vi "WFS_Thorlabs_testPanel.vi"() -> ()   [LabVIEW 2016]
uses:
  Type definitions/WFS cam and pupil config.ctl
  Type definitions/WFS wavefront and Zernike fit.ctl
  Type definitions/WFS wavefront data.ctl
  Type definitions/States enum in WFS_Thorlabs_testPanel.ctl
  <vilib>/Analysis/5stat.llb/RMS (DBL).vi
  <vilib>/Analysis/baseanly.llb/Mean (DBL).vi
  <vilib>/Platform/NI_3dgraph.lvlib
  <vilib>/Analysis/NI_AALBase.lvlib
  <vilib>/Analysis/NI_AALPro.lvlib
panel:
  in  "Rolling average, frames":i32=10 caption="Average Count" min=1 max=255 step=1
  in  "Output":enum32{"Graphical output", "Numerical"}(tab)
  in  "Measured WF":refnum<k7>(container)
  out "Zernike coeffs":dbl[](graph)
  in  "Fitting errors":refnum<k7>(container)
  out "WF data":T1
  out "Rad. of curvature (mm)":dbl
  out "error out":errorcluster
  out "spots_y":i32
  out "spots_x":i32
  out "Exp Time Incr":dbl=0.0554 caption="Exposure Time Incr"
  out "Exp time Max, ms":dbl=66.6147666666 caption="Exposure Time Max"
  out "Exp time Min, ms":dbl=0.07936666666666665 caption="Exposure Time Min"
  in  "stop":bool
  out "Ambient light":string
  out "Light power":string
  in  "WF and Zernike fit config":T2={"Limit meas. to pupil"=1, "Cancel WF tilt"=enum."Yes", "Zern. order max."=5, "wavelength, um"=0.633} {"wavelength, um" format="%.3f"; "Limit meas. to pupil" items=["Yes"=1, "No"=0]}
  in  "WFS cam & pupil config":T3={"Trigger Mode"=enum."Continuous", "Auto exposure"=TRUE, "Exposure time (ms)"=0.07936666666666667, "Master gain"=1.0, "Cam img size"=1, "Pupil diam X (mm)"=4.5, "Pupil diam Y (mm)"=4.5} {"Cam img size" items=["1280x1024 = 5.95x4.76mm", "1024x1024 = 4.76x4.76mm", "768x768 = 3.57x3.57mm", "512x512 = 2.38x2.38mm", "320x320 = 1.49x1.49mm"]; "Exposure time (ms)" min=0.0793667 max=66.6148 step=0.0554 format="%#.6f"}
  in  "error in":errorcluster
  out "InstName":string caption="Instrument Name"
  # "Shack-Hartmann wavefront sensor config"
  # "All units are lambda (wavelength)"
  # "For Shack-Hartmann sensor models:\nThorlabs WFS-150, WFS-300, WFS-20"
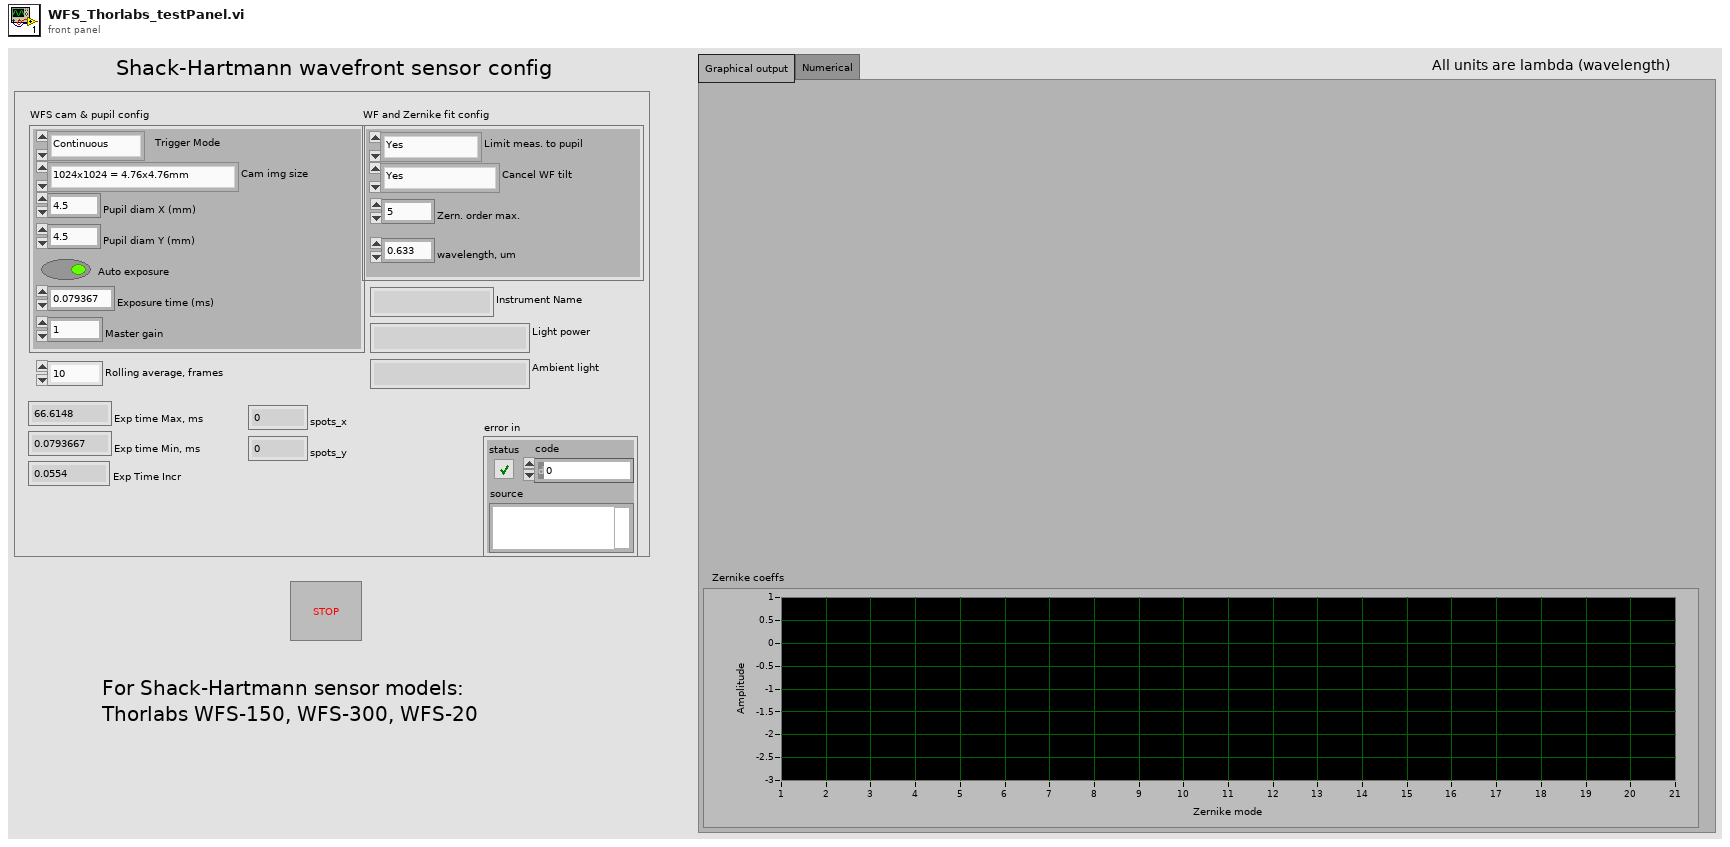
[diagram p1: front panel]
types:
  T1 = typedef "WFS wavefront data.ctl" = cluster{"ArrayWF":sgl[][], "ArrayZernike":sgl[], "WF_PV":dbl, "WF_RMS":dbl, "FittingErrors":dbl[][], "Error_mean":dbl, "Error_RMS":dbl}
  T2 = typedef "WFS wavefront and Zernike fit.ctl" = cluster{"Limit meas. to pupil":i32, "Cancel WF tilt":enum16{"No", "Yes"}, "Zern. order max.":i32, "wavelength, um":dbl}
  T3 = typedef "WFS cam and pupil config.ctl" = cluster{"Trigger Mode":enum16{"Continuous", "Slope H->L", "Slope L->H", "Software"}, "Auto exposure":bool, "Exposure time (ms)":dbl, "Master gain":dbl, "Cam img size":i32, "Pupil diam X (mm)":dbl, "Pupil diam Y (mm)":dbl}
  T4 = typedef "States enum in WFS_Thorlabs_testPanel.ctl" = enum16{"Initialize", "Configure", "Measure", "Stop", "Exit", "Health check"}
  T5 = enum16{"Initialize", "Configure", "Measure", "Stop", "Exit"}
  T6 = enum16{"Initialize", "Configure", "Measure", "Stop", "Exit", "Health check"}
  T7 = enum16{"Continuous", "Slope H->L", "Slope L->H", "Software"}
  T8 = cluster{"ArrayWF":dbl[][], "ArrayZernike":dbl[], "WF_PV":dbl, "WF_RMS":dbl, "FittingErrors":dbl[][], "Error_mean":dbl, "Error_RMS":dbl}
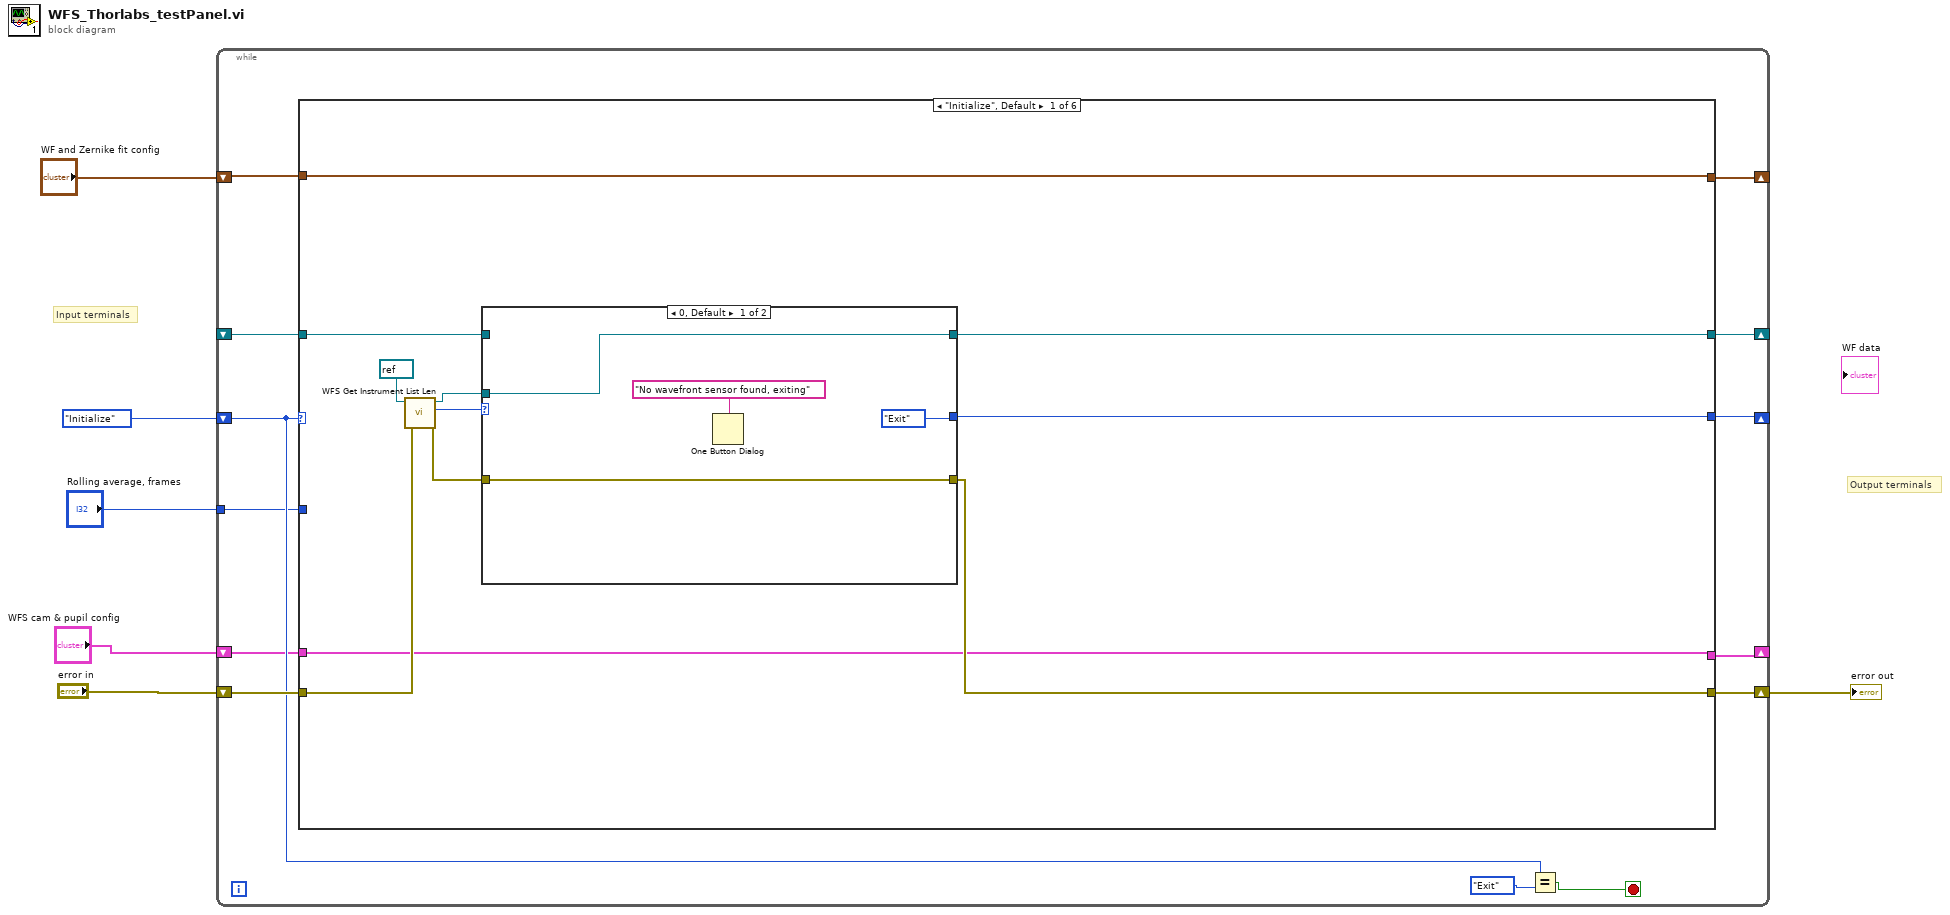
[diagram p0: block diagram]
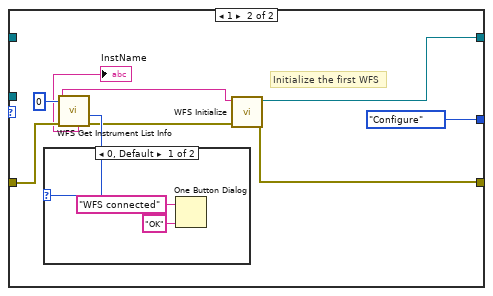
[diagram p2: hidden frame]
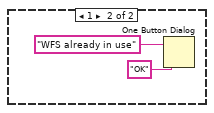
[diagram p3: hidden frame]
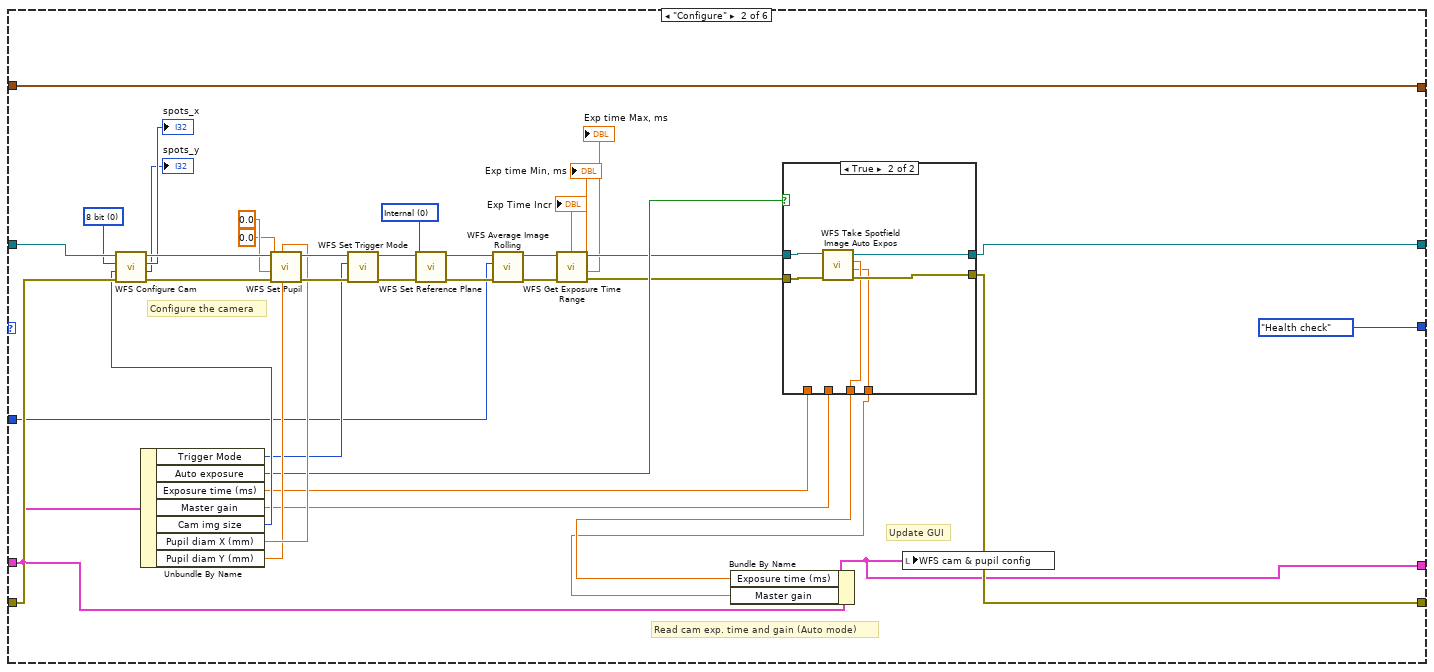
[diagram p4: hidden frame]
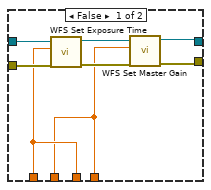
[diagram p5: hidden frame]
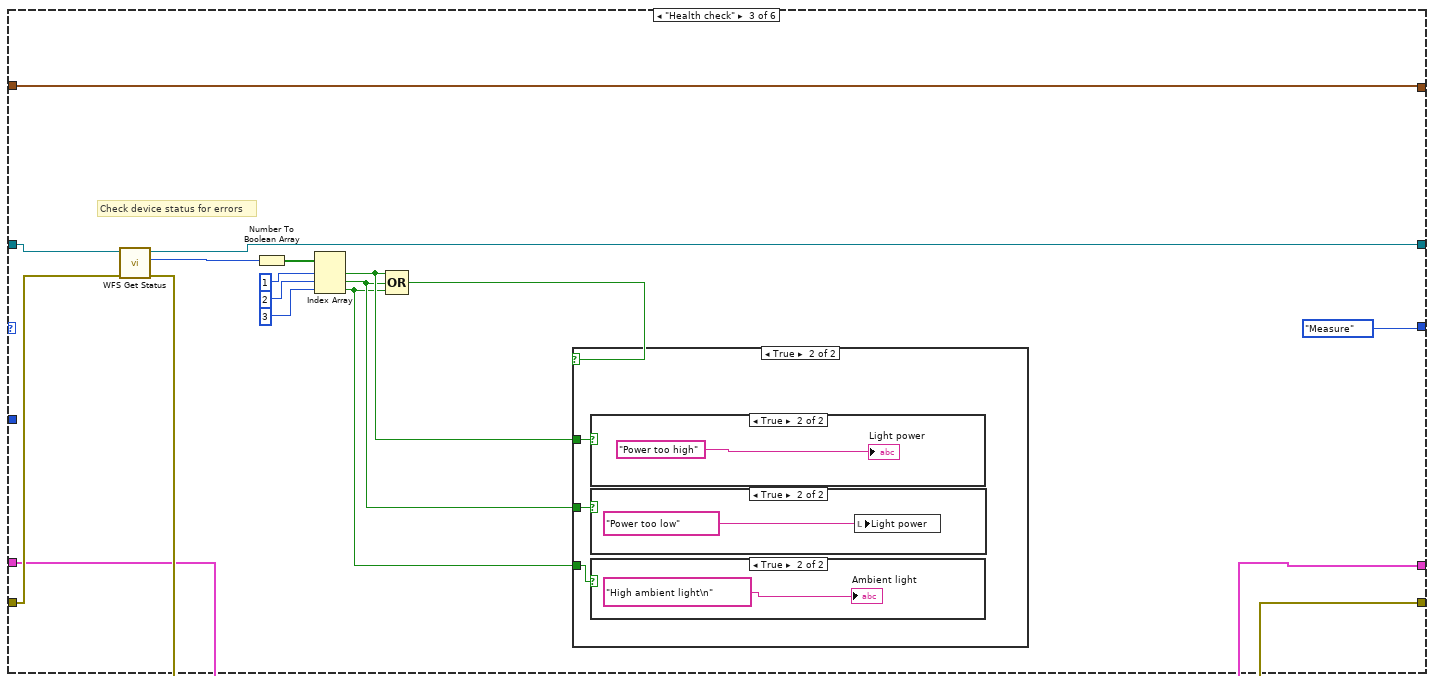
[diagram p6: hidden frame]
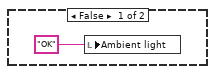
[diagram p8: hidden frame]
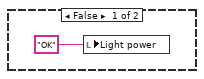
[diagram p9: hidden frame]
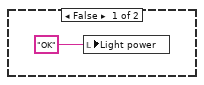
[diagram p10: hidden frame]
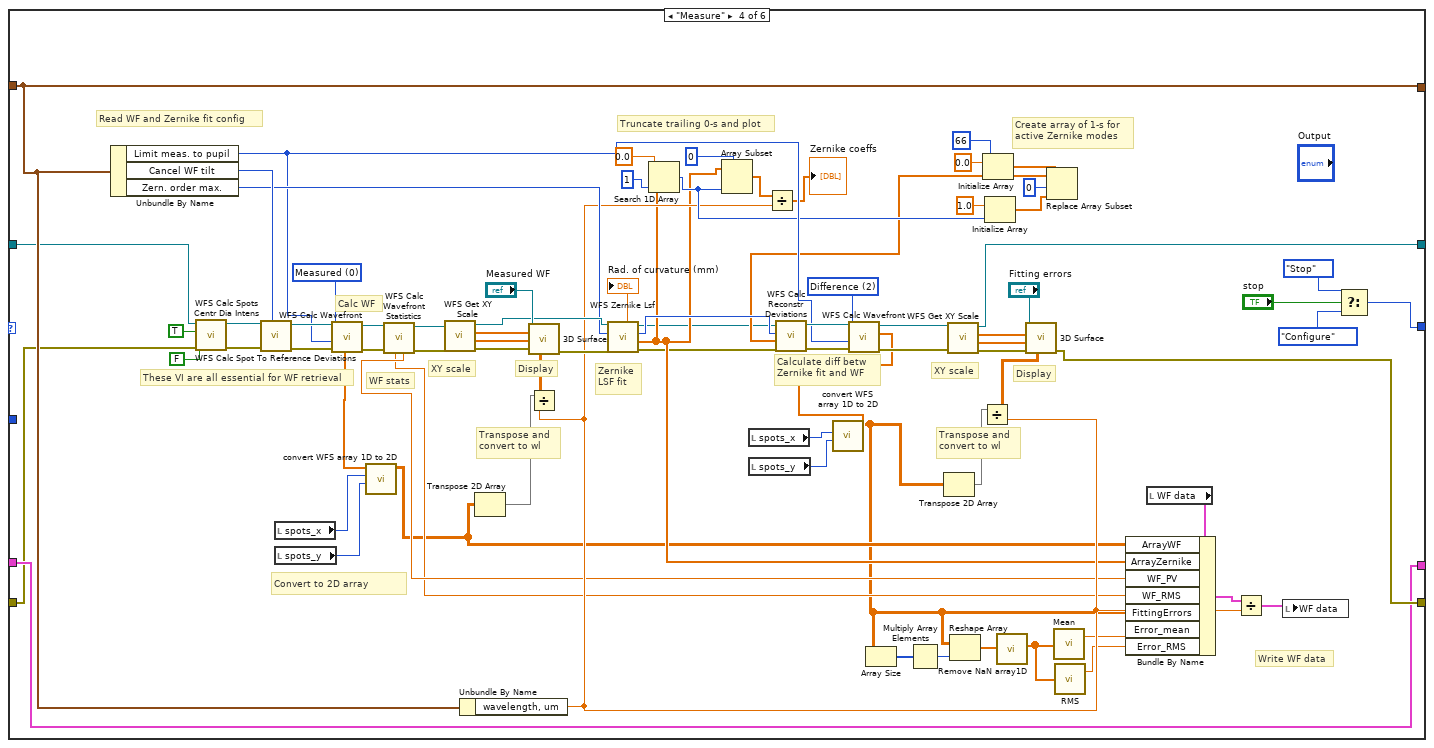
[diagram p11: hidden frame]
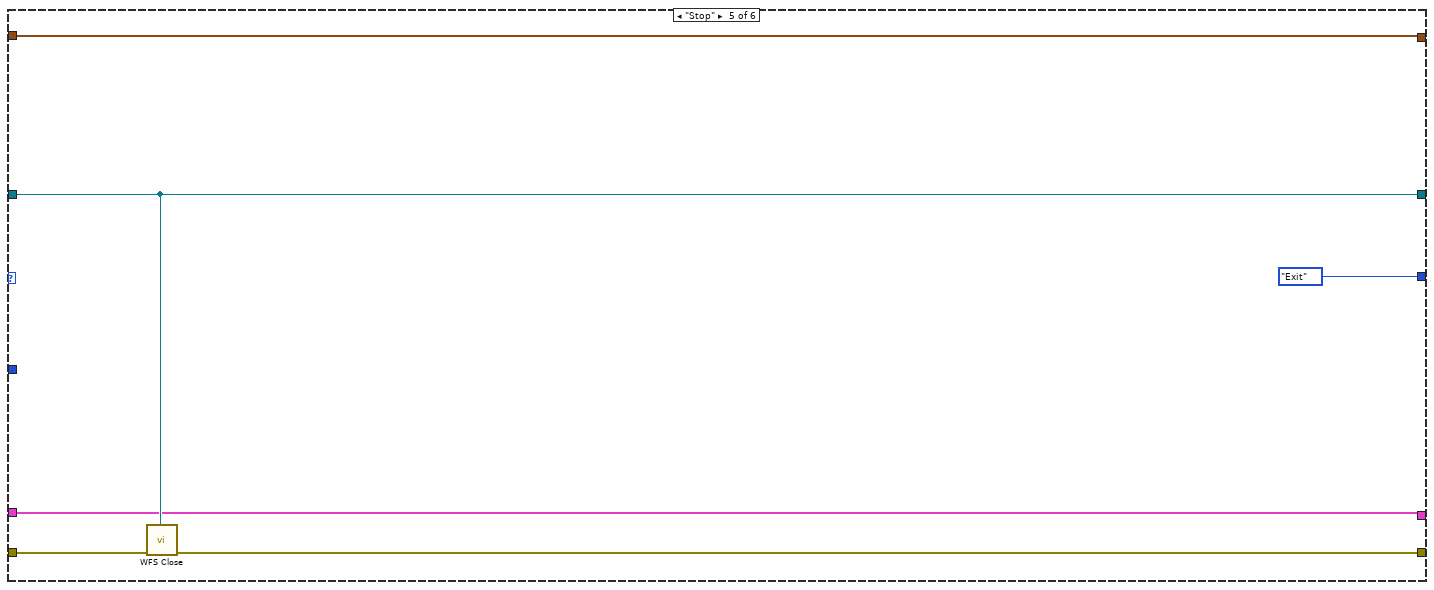
[diagram p12: hidden frame]
diagram:
  # "Input terminals"
  # "Output terminals"
  n1 = while {
    shift-right: [w18] -> w2
    shift-left: "error in" -> [w19]
    shift-right: [w17] -> _
    shift-left: _ -> [w16]
    shift-right: [w15] -> _
    shift-left: States_enum_in_WFS_Thorlabs_testPanel."Initialize" -> [w14]
    shift-right: [w10] -> _
    shift-left: "WFS cam & pupil config" -> [w11]
    shift-right: [w8] -> _
    shift-left: "WF and Zernike fit config" -> [w9]
    tunnel: "Rolling average, frames" -> [w7]
    stop <- w13 stop-if-true
    n2 = case shown="\"Initialize\", Default" w14 {
      selector: w14 -> [_ _ _ _ _ w213]
      tunnel: w19 -> [w30 w85 w111 w127 w211 w215]
      tunnel: [w26 w79 w104 w171 w210 w215] -> w18
      tunnel: [w25 w80 w109 w174 w212 w216] -> w17
      tunnel: w16 -> [w24 w86 w112 w126 w212 w216]
      tunnel: [w21 T6."Health check" T5."Measure" w189 T6."Exit" w213] -> w15
      tunnel: w11 -> [w23 w65 w103 w128 w209 w214]
      tunnel: [w23 w64 w103 w128 w209 w214] -> w10
      tunnel: w9 -> [w22 w56 w102 w157 w208 w217]
      tunnel: [w22 w56 w102 w157 w208 w217] -> w8
      tunnel: w7 -> [_ w48 _ _ _ _]
      frame "Initialize", Default {
        n3 = call "WFS Get Instrument List Len.vi"("error in (no error)"=w30, "instrument handle"=refnum<visa-resource-name> refnum) -> ("error out"=w27:errorcluster, "Instrument Count"=w28:i32, "instrument handle out"=w20:refnum<visa-resource-name>)  [unwired: 7 in]
        n4 = case shown="0, Default" w28 {
          tunnel: [w33 w38] -> w26
          tunnel: w27 -> [w33 w42]
          tunnel: [w31 w39] -> w25
          tunnel: w24 -> [_ _]
          tunnel: [T5."Exit" T5."Configure"] -> w21
          tunnel: w20 -> [w31 _]
          frame 0, Default {
            n5 = One Button Dialog(message="No wavefront sensor found, exiting") -> ()  [unwired: 1 in, 1 out]
          }
          frame 1 {
            # "Initialize the first WFS"
            n6 = call "WFS Get Instrument List Info.vi"("error in (no error)"=w42, "Instrument List Index"=0) -> ("error out"=w40:errorcluster, "In Use"=w41:i32, "Instrument Name"=→"InstName":string, "Resource Name"=w37:string)  [unwired: 3 in, 3 out]
            n7 = case shown="0, Default" w41 {
              frame 0, Default {
                n8 = One Button Dialog(message="WFS connected", button name ("OK")="OK") -> ()  [unwired: 1 out]
              }
              frame 1 {
                n9 = One Button Dialog(message="WFS already in use", button name ("OK")="OK") -> ()  [unwired: 1 out]
              }
            }
            n10 = call "WFS Initialize.vi"("error in (no error)"=w40, "resource name"=w37) -> ("error out"=w38:errorcluster, "instrument handle out"=w39:refnum<visa-resource-name>)  [unwired: 8 in]
          }
        }
      }
      frame "Configure" {
        w73 = 0 items=["Internal", "User"] ("Reference Index (Internal)")
        w76 = 0 items=["16 bit"=1, "8 bit"=0] ("Pixel Format (8 bit)")
        # "Update GUI"
        # "Read cam exp. time and gain (Auto mode)"
        # "Configure the camera"
        n11 = Unbundle By Name(w65) -> ("Trigger Mode"=w69:T7, "Auto exposure"=w68:bool, "Exposure time (ms)"=w67:dbl, "Master gain"=w66:dbl, "Cam img size"=w72:i32, "Pupil diam X (mm)"=w71:dbl, "Pupil diam Y (mm)"=w70:dbl)
        n12 = call "WFS Configure Cam.vi"("error in (no error)"=w85, "Cam Resol. Index (1280x1024      640x480      1440x1080)"=w72, "Pixel Format (8 bit)"=w76, "instrument handle"=w86) -> ("error out"=w84:errorcluster, "Spots Y"=→"spots_y":i32, "Spots X"=→"spots_x":i32, "instrument handle out"=w83:refnum<visa-resource-name>)  [unwired: 4 in]
        n13 = call "WFS Set Pupil.vi"("Pupil Diameter Y mm"=w70, "Pupil Diameter X mm"=w71, "error in (no error)"=w84, "Pupil Center Y mm"=0.0, "Pupil Center X mm"=0.0, "instrument handle"=w83) -> ("error out"=w81:errorcluster, "instrument handle out"=w82:refnum<visa-resource-name>)  [unwired: 4 in]
        n14 = call "WFS Set Trigger Mode.vi"("error in (no error)"=w81, "Trigger Mode"=w69, "instrument handle"=w82) -> ("error out"=w74:errorcluster, "instrument handle out"=w75:refnum<visa-resource-name>)  [unwired: 7 in]
        n15 = call "WFS Set Reference Plane.vi"("error in (no error)"=w74, "Reference Index (Internal)"=w73, "instrument handle"=w75) -> ("error out"=w49:errorcluster, "instrument handle out"=w50:refnum<visa-resource-name>)  [unwired: 7 in]
        n16 = call "WFS Average Image Rolling.vi"("error in (no error)"=w49, "Average Count"=w48, "instrument handle"=w50) -> ("error out"=w51:errorcluster, "instrument handle out"=w52:refnum<visa-resource-name>)  [unwired: 7 in]
        n17 = call "WFS Get Exposure Time Range.vi"("error in (no error)"=w51, "instrument handle"=w52) -> ("error out"=w60:errorcluster, "Exposure Time Max"=→"Exp time Max, ms":dbl, "Exposure Time Min"=→"Exp time Min, ms":dbl, "instrument handle out"=w61:refnum<visa-resource-name>, "Exposure Time Incr"=→"Exp Time Incr":dbl)  [unwired: 5 in]
        n18 = case shown="True" w68 {
          tunnel: [w92 w100] -> w80
          tunnel: [w91 w99] -> w79
          tunnel: w60 -> [w90 w97]
          tunnel: w61 -> [w89 w98]
          tunnel: w67 -> [w88 _]
          tunnel: w66 -> [w87 _]
          tunnel: [w88 w96] -> w63
          tunnel: [w87 w95] -> w62
          frame False {
            n19 = call "WFS Set Exposure Time.vi"("error in (no error)"=w90, "Exposure Time Set"=w88, "instrument handle"=w89) -> ("error out"=w94:errorcluster, "instrument handle out"=w93:refnum<visa-resource-name>)  [unwired: 6 in, 1 out]
            n20 = call "WFS Set Master Gain.vi"("error in (no error)"=w94, "Master Gain Set"=w87, "instrument handle"=w93) -> ("error out"=w91:errorcluster, "instrument handle out"=w92:refnum<visa-resource-name>)  [unwired: 6 in, 1 out]
          }
          frame True {
            n21 = call "WFS Take Spotfield Image Auto Expos.vi"("error in (no error)"=w97, "instrument handle"=w98) -> ("error out"=w99:errorcluster, "Master Gain Act"=w95:dbl, "Exposure Time Act"=w96:dbl, "instrument handle out"=w100:refnum<visa-resource-name>)  [unwired: 6 in]
          }
        }
        n22 = Bundle By Name(cluster=w65, "Exposure time (ms)"=w63, "Master gain"=w62) -> (w64:T3)
        n23 = local write "WFS cam & pupil config"(w64) -> ()
      }
      frame "Health check" {
        # "Check device status for errors"
        n24 = call "WFS Get Status.vi"("error in (no error)"=w111, "instrument handle"=w112) -> ("error out"=w104:errorcluster, "Device Status"=w110:i32, "instrument handle out"=w109:refnum<visa-resource-name>)  [unwired: 7 in]
        n25 = Number To Boolean Array(number=w110) -> (Boolean array=w113:bool[])
        n26 = Index Array(array=w113, index #1=1 ("index"), index #2=2 ("index"), index #3=3 ("index")) -> (element #1=w107:bool, element #2=w106:bool, element #3=w105:bool)
        n27 = Compound Arithmetic op=OR(w107, w106, w105) -> (w108:bool)
        n28 = case shown="True" w108 {
          tunnel: w107 -> [_ w119]
          tunnel: w106 -> [_ w118]
          tunnel: w105 -> [_ w117]
          frame False {
          }
          frame True {
            n29 = case shown="True" w119 {
              frame False {
                n30 = local write "Light power"("OK" ("Device Status")) -> ()
              }
              frame True {
                "Light power" <- "Power too high"
              }
            }
            n31 = case shown="True" w118 {
              frame False {
                n32 = local write "Light power"("OK" ("Device Status")) -> ()
              }
              frame True {
                n33 = local write "Light power"("Power too low") -> ()
              }
            }
            n34 = case shown="True" w117 {
              frame False {
                n35 = local write "Ambient light"("OK" ("Device Status 2")) -> ()
              }
              frame True {
                "Ambient light" <- "High ambient light\n"
              }
            }
          }
        }
      }
      frame "Measure" {
        w180 = 2 items=["Measured", "Reconstructed", "Difference"] ("Wavefront Type (Measured)")
        w185 = 0 items=["Measured", "Reconstructed", "Difference"] ("Wavefront Type (Measured)")
        # "Create array of 1-s for \nactive Zernike modes"
        # "Truncate trailing 0-s and plot"
        # "Transpose and \nconvert to wl"
        # "Transpose and \nconvert to wl"
        # "Convert to 2D array"
        # "Display"
        # "XY scale"
        # "Calculate diff betw \nZernike fit and WF"
        # "Write WF data"
        # "Calc WF"
        # "XY scale"
        # "WF stats"
        # "Display"
        # "Read WF and Zernike fit config"
        # "These VI are all essential for WF retrieval"
        # "Zernike \nLSF fit"
        n36 = Unbundle By Name(w157) -> ("Limit meas. to pupil"=w179:i32, "Cancel WF tilt"=w194:enum16{"No", "Yes"}, "Zern. order max."=w184:i32)
        n37 = call "WFS Calc Spots Centr Dia Intens.vi"("error in (no error)"=w127, "Calculate Diameters (Off)"=FALSE, "Dynamic Noise Cut (On)"=TRUE, "instrument handle"=w126) -> ("error out"=w199:errorcluster, "instrument handle out"=w200:refnum<visa-resource-name>)  [unwired: 6 in]
        n38 = call "WFS Calc Spot To Reference Deviations.vi"("error in (no error)"=w199, "Cancel Wavefront Tilt (No)"=w194, "instrument handle"=w200) -> ("error out"=w198:errorcluster, "instrument handle out"=w197:refnum<visa-resource-name>)  [unwired: 7 in]
        n39 = local read "spots_x"() -> (w141:i32)
        n40 = local read "spots_y"() -> (w140:i32)
        n41 = call "WFS Calc Wavefront.vi"("error in (no error)"=w198, "Limit to Pupil (No)"=w179, "Wavefront Type (Measured)"=w185, "instrument handle"=w197) -> ("error out"=w133:errorcluster, "Array Wavefront"=w142:sgl[], "instrument handle out"=w134:refnum<visa-resource-name>)  [unwired: 5 in]
        n42 = call "convert WFS array 1D to 2D.vi"("spots_y"=w140, "spots_x"=w141, "WF 1D input"=w142) -> ("FW 2D output"=w139:sgl[][])  [unwired: 8 in]
        n43 = call "WFS Calc Wavefront Statistics.vi"("error in (no error)"=w133, "instrument handle"=w134) -> ("error out"=w131:errorcluster, "instrument handle out"=w132:refnum<visa-resource-name>, "Diff"=w150:dbl, "RMS"=w149:dbl)  [unwired: 2 in, 4 out]
        n44 = call "WFS Get XY Scale.vi"("error in (no error)"=w131, "instrument handle"=w132) -> ("error out"=w206:errorcluster, "Array Scale Y"=w204:sgl[], "Array Scale X"=w205:sgl[], "instrument handle out"=w196:refnum<visa-resource-name>)  [unwired: 6 in]
        n45 = Unbundle By Name(w157) -> ("wavelength, um"=w152:dbl)
        n46 = Transpose 2D Array(2D array=w139) -> (transposed array=w187:sgl[][])
        n47 = Divide(x=w187, y=w152) -> (x/y=w186:dbl[][])
        n48 = call <vilib>:"3D Surface.vi"("z matrix"=w186, "error in (no error)"=w206, "y vector"=w204, "x vector"=w205, "3D graph"="Measured WF") -> ("error out"=w195:errorcluster)  [unwired: 5 in, 1 out]
        n49 = call "WFS Zernike Lsf.vi"("error in (no error)"=w195, "Zernike Orders In"=w184, "instrument handle"=w196) -> ("error out"=w129:errorcluster, "Array Zernike um"=w151:sgl[], "Zernike Orders Out"=w183:i32, "instrument handle out"=w130:refnum<visa-resource-name>, "RoC mm"=→"Rad. of curvature (mm)":dbl)  [unwired: 3 in, 1 out]
        n50 = Search 1D Array(1D array=w151, element=sgl 0.0, start index (0)=1) -> (index of element=w161:i32)
        n51 = Array Subset(array=w151, index=0, length=w161) -> (w156:sgl[])
        n52 = local read "spots_x"() -> (w138:i32)
        n53 = local read "spots_y"() -> (w137:i32)
        n54 = Divide(x=w156, y=w152) -> (x/y=→"Zernike coeffs":dbl[])
        n55 = Initialize Array(0.0 ("element"), 66 ("dimension size")) -> (w163:dbl[])
        n56 = Initialize Array(1.0 ("element"), w161) -> (w159:dbl[])
        n57 = Replace Array Subset(array=w163, new element=w159, index=0) -> (w158:dbl[])
        n58 = call "WFS Calc Reconstr Deviations.vi"("error in (no error)"=w129, "Array Zernike Reconstruct"=w158, "Zernike Orders"=w183, "instrument handle"=w130) -> ("error out"=w182:errorcluster, "instrument handle out"=w181:refnum<visa-resource-name>)  [unwired: 4 in, 2 out]
        n59 = call "WFS Calc Wavefront.vi"("error in (no error)"=w182, "Limit to Pupil (No)"=w179, "Wavefront Type (Measured)"=w180, "instrument handle"=w181) -> ("error out"=w176:errorcluster, "Array Wavefront"=w136:sgl[], "instrument handle out"=w175:refnum<visa-resource-name>)  [unwired: 5 in]
        n60 = call "convert WFS array 1D to 2D.vi"("spots_y"=w137, "spots_x"=w138, "WF 1D input"=w136) -> ("FW 2D output"=w135:sgl[][])  [unwired: 8 in]
        n61 = Array Size(array=w135) -> (size(s)=w147:i32[])
        n62 = Multiply Array Elements(1:w147) -> (0:w148:i32)
        n63 = Transpose 2D Array(2D array=w135) -> (transposed array=w170:sgl[][])
        n64 = call "WFS Get XY Scale.vi"("error in (no error)"=w176, "instrument handle"=w175) -> ("error out"=w177:errorcluster, "Array Scale Y"=w172:sgl[], "Array Scale X"=w173:sgl[], "instrument handle out"=w174:refnum<visa-resource-name>)  [unwired: 6 in]
        n65 = Reshape Array(w135, w148) -> (w144:sgl[])
        n66 = Divide(x=w170, y=w152) -> (x/y=w169:dbl[][])
        n67 = call "Remove NaN array1D.vi"("Array in"=w144) -> ("Array out"=w143:dbl[])  [unwired: 10 in]
        n68 = call <vilib>:"3D Surface.vi"("z matrix"=w169, "error in (no error)"=w177, "y vector"=w172, "x vector"=w173, "3D graph"="Fitting errors") -> ("error out"=w171:errorcluster)  [unwired: 5 in, 1 out]
        n69 = call-poly <vilib>:"Mean.vi"("X"=w143) -> ("mean"=w145:dbl)  [unwired: 1 out]
        n70 = call-poly <vilib>:"RMS.vi"("X"=w143) -> ("rms value"=w146:dbl)  [unwired: 1 out]
        n71 = local read "WF data"() -> (w193:T1)
        n72 = Bundle By Name(cluster=w193, "ArrayWF"=w139, "ArrayZernike"=w151, "WF_PV"=w150, "WF_RMS"=w149, "FittingErrors"=w135, "Error_mean"=w145, "Error_RMS"=w146) -> (w154:T1)
        n73 = Divide(x=w154, y=w152) -> (x/y=w153:T8)
        n74 = local write "WF data"(w153) -> ()
        n75 = Select(t=T5."Stop", s="stop", f=T5."Configure") -> (s? t:f=w189:T5)
      }
      frame "Stop" {
        n76 = call "WFS Close.vi"("error in (no error)"=w211, "instrument handle"=w212) -> ("error out"=w210:errorcluster)  [unwired: 9 in]
      }
      frame "Exit" {
      }
    }
    n77 = Equal?(x=w14, y=T5."Exit") -> (x = y?=w13:bool)
  }
  "error out" <- w2
